vi "MathCad_Matrix_Get_1D.vi"(0 "Worksheet Reference":refnum<k7>, 1 "Mathcad.IMatrixValue Refnum":refnum<k7>, 2 "error in":errorcluster) -> (3 "Worksheet Reference Out":refnum<k7>, 4 "Mathcad.IMatrixValue Refnum":refnum<k7>, 5 "Array":dbl[](array[numeric]) format="%.2f", 6 "error out":errorcluster)   [LabVIEW 2015]
doc: "Gets the value from the reference retrieved from the getrefnum VI."
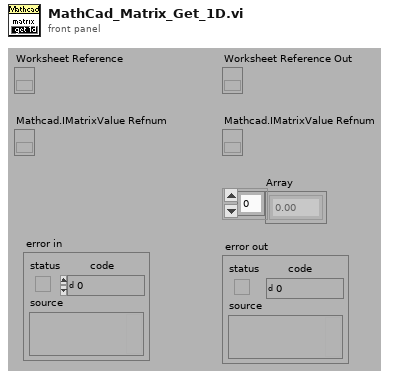
[diagram p1: front panel]
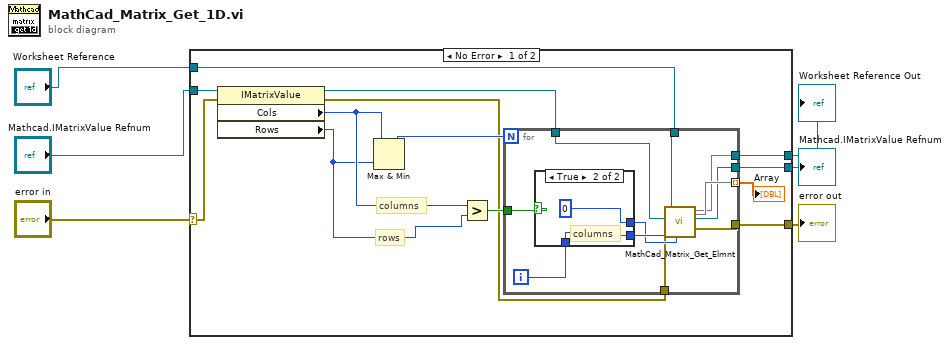
[diagram p0: block diagram]
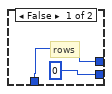
[diagram p2: hidden frame]
diagram:
  n1 = case shown="No Error" "error in" {
    selector: "error in" -> [w13 w35]
    tunnel: "Mathcad.IMatrixValue Refnum" -> [w18 w36]
    tunnel: "Worksheet Reference" -> [w9 w37]
    tunnel: [w8 w37] -> w3
    tunnel: [w11 w35] -> w4
    tunnel: [w7 w36] -> w5
    frame No Error {
      # "rows"
      # "columns"
      n2 = property class="IMatrixValue"(reference=w18, error in=w13) -> (reference out=w16:refnum<k7>, error out=w12:errorcluster, "Cols"=w15:i32, "Rows"=w14:i32)
      n3 = Max & Min(x=w15, y=w14) -> (max(x,y)=w19:i32)  [unwired: 1 out]
      n4 = Greater?(x=w15, y=w14) -> (0:w17:bool)
      n5 = for {
        N: w19 -> [_]
        tunnel: w17 -> [w30]
        tunnel: w16 -> [w29]
        tunnel: w12 -> [w23]
        tunnel: [w27] -> w11
        tunnel: [w26] -> w10 mode=indexing
        tunnel: w9 -> [w22]
        tunnel: [w21] -> w8
        tunnel: [w20] -> w7
        i -> [w28]
        n6 = case shown="True" w30 {
          tunnel: w28 -> [w31 w34]
          tunnel: [0 w34] -> w25
          tunnel: [w31 0] -> w24
          frame False {
            # "rows"
          }
          frame True {
            # "columns"
          }
        }
        n7 = call "MathCad_Matrix_Get_Elmnt.vi"("row"=w24, "col"=w25, "error in"=w23, "Mathcad.IMatrixValue Refnum"=w29, 9:w22) -> ("error out"=w27:errorcluster, "Mathcad.IMatrixValue Refnum"=w20:refnum<k7>, 3:w21, 5:w26)  [unwired: 1 out]
      }
      "Array" <- w10
    }
    frame Error {
    }
  }
  "Mathcad.IMatrixValue Refnum" <- w5
  "error out" <- w4
  "Worksheet Reference Out" <- w3
